vi "Whirlybird FPGA Main.vi"() -> (3 "Roll":i16)   [LabVIEW 2012]
uses:
  FPGA Samples/spi_single port_example/FPGA/Controls/FPGA SPI_Cmd.ctl
  <vilib>/Platform/TimedLoop/XDataNode/timing_clust.ctl
  <vilib>/Platform/TimedLoop/XDataNode/nitl_modes.ctl
  <vilib>/Platform/TimedLoop/XDataNode/wakeup.ctl
  FPGA Samples/spi_single port_example/FPGA/Controls/FPGA SPI_Arb Loop State.ctl
  <vilib>/rvi/eio/common/nirviEmuTemplateMethod_errors.vi
  <vilib>/rvi/Emulation/niFpgaSctlEmulationGetInTimedLoop.vi
  <vilib>/rvi/Emulation/niFpgaSctlEmulationGlobalWrite.vi
  FPGA Samples/spi_single port_example/FPGA/Code/FPGA SPI_Globals.vi
  <vilib>/rvi/DataTransferAndStorage/Container/Common/niFpgaContainerGetUniqueNameForEmu.vi
  <vilib>/rvi/FIFO/Fifo_Resource/nirvififoEmulationSetSize.vi
  <vilib>/rvi/errors/niFpgaSetErrorForExecOnDevCompSimple.vi
  <vilib>/rvi/eio/common/nirviEmuReportErrorAndStop.vi
  <vilib>/rvi/Emulation/niFpgaSctlEmulationFifoFullMgr.vi
  <vilib>/rvi/Emulation/niFpgaSctlEmulationResourceMgr.vi
  <vilib>/rvi/Emulation/niFpgaSctlEmulationRegisterWithScheduler.vi
  <vilib>/rvi/Emulation/niFpgaSctlEmulationScheduler.vi
  <vilib>/Platform/TimedLoop/XDataNode/XDataNode.xnode
  <vilib>/eio/EIONode/EIONode.xnode
  <vilib>/eio/EIOMethodNode/EIOMethodNode.xnode
  <vilib>/rvi/DataTransferAndStorage/Container/XNode/niFpgaContainer.xnode
  <vilib>/rvi/FIFO/Fifo_Resource/nirvififoEmulationWrite.vi
  <vilib>/rvi/FIFO/Fifo_Resource/nirvififoEmulationRead.vi
  <vilib>/Platform/TimedLoop/XDataNode/XDNodeRunTimeDep.lvlib
panel:
  in  "Auto Zero?":bool
  in  "IMU Reset":bool=TRUE
  in  "SPI_Ack Read":bool
  out "SPI_Read Flag":bool
  out "SPI_Read Data":u8
  in  "SPI_Write Data":u8
  in  "SPI_Write Flag":bool
  in  "SPI_Total Bytes":u16=1
  in  "SPI_Total Bits":u16=8
  in  "SPI_CS":u8=1 format="%08b"
  in  "SPI_CS Active State":bool caption="SPI_CS\nActive State"
  in  "SPI_Clock Divider":u32=20
  in  "SPI_CPHA":bool
  in  "SPI_CPOL":bool
  in  "SPI_Cmd":T1=enum."Configure"
  in  "SPI_Port":u8
  in  "SPI_Start":bool
  out "Ready":bool
  in  "MC2":u32(slide)=20 step=546002432 scale=0.0..600.0
  in  "MC1":u32(slide)=20 scale=0.0..600.0
  out "Pitch":i16
  out "Yaw":i16
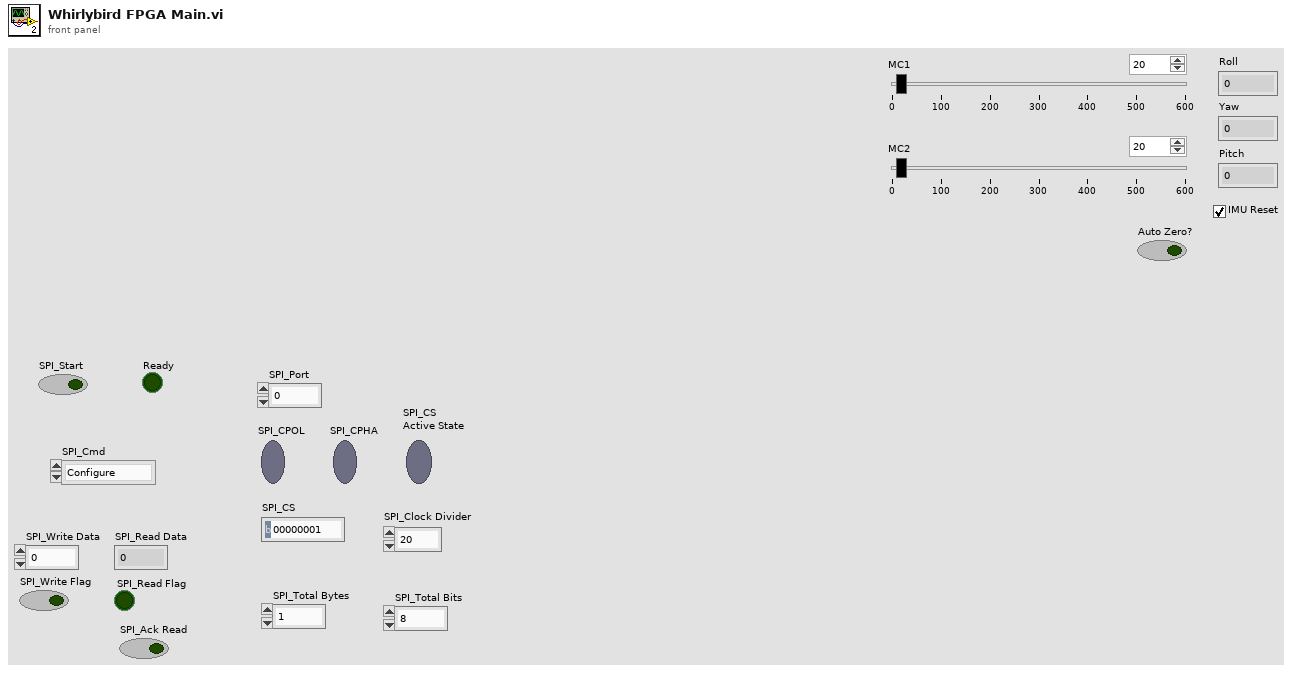
[diagram p1: front panel]
types:
  T1 = typedef "FPGA SPI_Cmd.ctl" = enum8{"Idle", "Write/Read SPI", "Configure"}
  T2 = cluster{"SCLK":refnum<k21>, "CS_1":refnum<k21>, "MOSI":refnum<k21>, "MISO":refnum<k21>, "CS_2":refnum<k21>}
  T3 = typedef "FPGA SPI_Arb Loop State.ctl" = enum8{"Idle", "Init", "Write", "Start", "Read", "Wait Until Done"}
  T4 = typedef "XDNodeRunTimeDep.lvlib/timing_clust.ctl" = cluster{"Expected End [f-1]":u64, "Actual End [f-1]":u64, "Finished Late? [f-1]":bool, "Expected End [i-1]":u64, "Actual End [i-1]":u64, "Finished Late? [i-1]":bool, "Expected Start [i]":u64, "Actual Start [i]":u64, "Expected Start [f]":u64, "Actual Start [f]":u64, "Source Name":string, "Structure Name":string, "Period":i64, "Deadline":i64, "Offset":i64, "Start":i64, "Priority":i32, "Timeout":i32, "Mode":T5, "Wakeup Reason":T6, "Error":errorcluster, "Source Type":string, "Secondary Source Type":string, "Global End Time":u64, "Global Start Time":u64, "Frame Duration":u64, "Iteration Duration":u64, "Assigned CPU":i32, "I/O Scan Engine Mode":u32}
  T5 = typedef "XDNodeRunTimeDep.lvlib/nitl_modes.ctl" = enum32{"No Change", "Process missed periods, maintain original phase", "Discard missed periods, maintain original phase", "Process missed periods, ignore original phase", "Discard missed periods, ignore original phase"}
  T6 = typedef "XDNodeRunTimeDep.lvlib/wakeup.ctl" = enum32{"Normal", "Aborted", "Asynchronous wakeup", "Timing source error", "Timed loop error", "Timeout"}
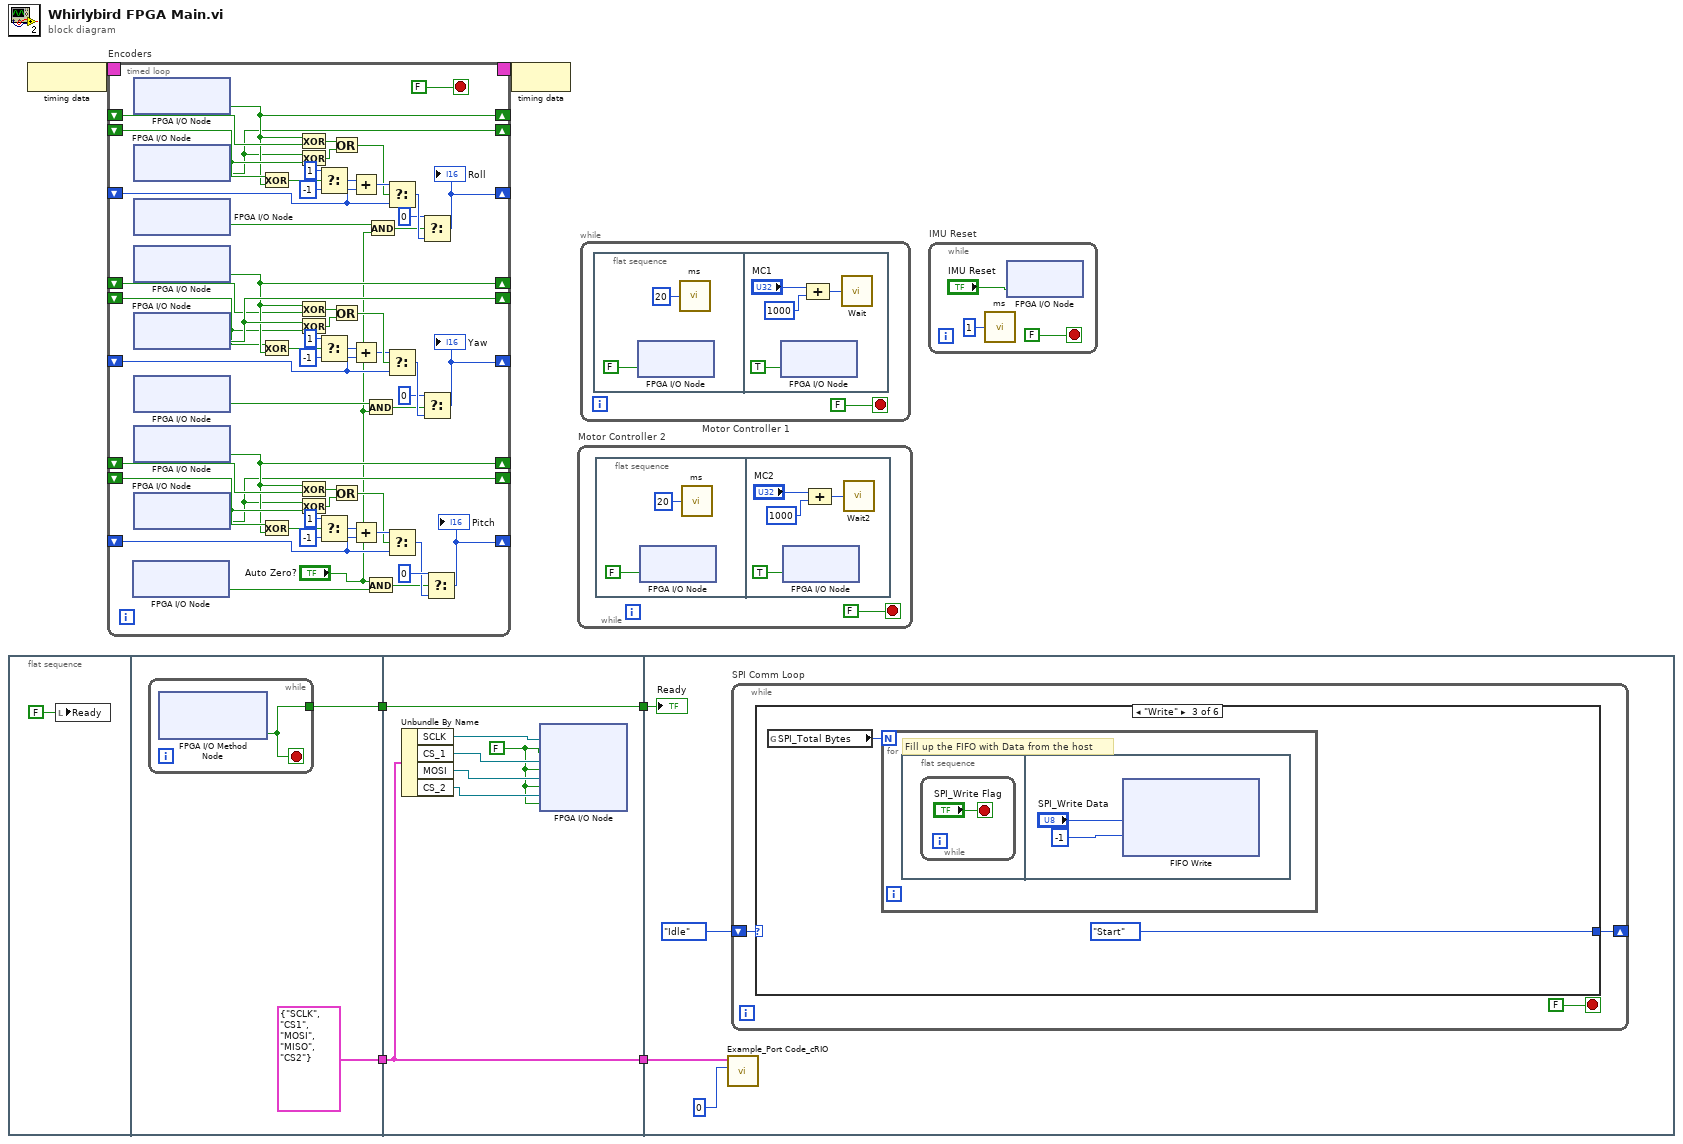
[diagram p0: block diagram]
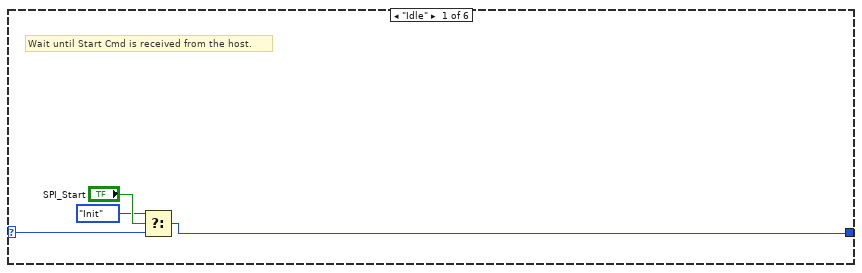
[diagram p2: hidden frame]
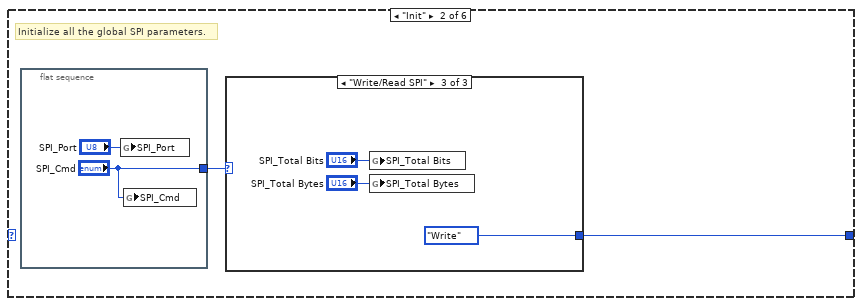
[diagram p3: hidden frame]
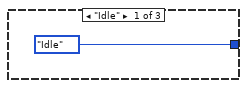
[diagram p4: hidden frame]
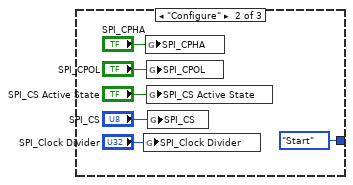
[diagram p5: hidden frame]
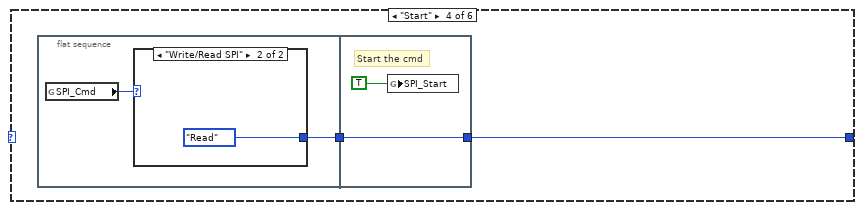
[diagram p6: hidden frame]
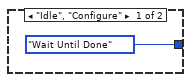
[diagram p7: hidden frame]
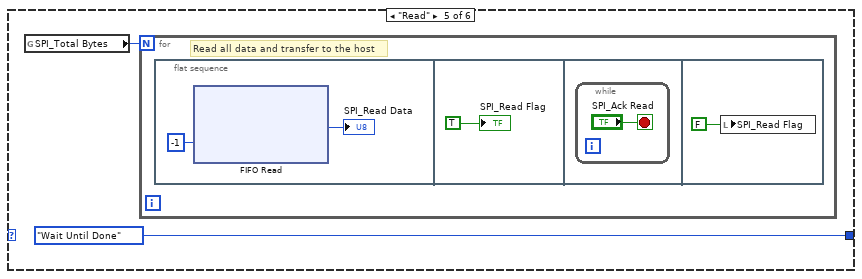
[diagram p8: hidden frame]
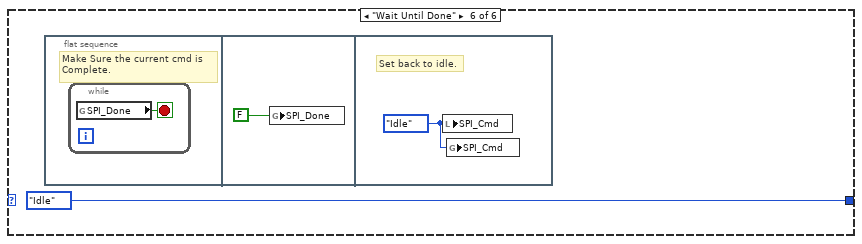
[diagram p9: hidden frame]
diagram:
  n1 = flat-sequence {
    tunnel: [T2 {"SCLK"="SCLK", "CS_1"="CS1", "MOSI"="MOSI", "MISO"="MISO", "CS_2"="CS2"} ("FPGA IO")] -> w4
    tunnel: [w8] -> w3
    tunnel: [w17] -> w2
    tunnel: w4 -> [w17]
    tunnel: [w13] -> w1
    tunnel: w3 -> [w13]
    tunnel: w2 -> [w19]
    tunnel: w1 -> [w18]
    frame #0 {
      n2 = local write "Ready"(FALSE ("Ready")) -> ()
    }
    frame #1 {
      n3 = while {
        tunnel: [w10] -> w8
        stop <- w10 stop-if-true
        n4 = xnode "FPGA I/O Method Node"() -> ("Ready"=w10:bool)  [unwired: 1 in, 1 out]
      }
    }
    frame #2 {
      w11 = FALSE ("I/O Item")
      n5 = Unbundle By Name(w17) -> ("SCLK"=w12:refnum<k21>, "CS_1"=w16:refnum<k21>, "MOSI"=w15:refnum<k21>, "CS_2"=w14:refnum<k21>)
      n6 = xnode "FPGA I/O Node"("I/O Item"=w11, "FPGA I/O In"=w12, "I/O Item"=w11, "FPGA I/O In"=w16, "I/O Item"=w11, "FPGA I/O In"=w15, "I/O Item"=w11, "FPGA I/O In"=w14) -> ()  [unwired: 4 out]
    }
    frame #3 {
      n7 = call "Example_Port Code_cRIO.vi"("Port"=i8 0, "FPGA IO"=w19) -> ()  [unwired: 10 out]
      n8 = while "SPI Comm Loop" {
        shift-right: [w23] -> _
        shift-left: FPGA_SPI_Arb_Loop_State."Idle" ("Action") -> [w22]
        stop <- FALSE stop-if-true
        n9 = case shown="\"Write\"" w22 {
          selector: w22 -> [w27 _ _ _ _ _]
          tunnel: [w25 w29 FPGA_SPI_Arb_Loop_State."Start" ("Action") w49 FPGA_SPI_Arb_Loop_State."Wait Until Done" ("Action") FPGA_SPI_Arb_Loop_State."Idle" ("Action")] -> w23
          frame "Idle" {
            # "Wait until Start Cmd is received from the host."
            n10 = Select(t=FPGA_SPI_Arb_Loop_State."Init" ("Action"), s="SPI_Start", f=w27) -> (s? t:f=w25:T3)
          }
          frame "Init" {
            # "Initialize all the global SPI parameters."
            n11 = flat-sequence {
              tunnel: ["SPI_Cmd"] -> w30
              frame #0 {
                n12 = global write "FPGA SPI_Globals.vi" "SPI_Port"("SPI_Port") -> ()
                n13 = global write "FPGA SPI_Globals.vi" "SPI_Cmd"("SPI_Cmd") -> ()
              }
            }
            n14 = case shown="\"Write/Read SPI\"" w30 {
              tunnel: [FPGA_SPI_Arb_Loop_State."Idle" ("Action") FPGA_SPI_Arb_Loop_State."Start" ("Action") FPGA_SPI_Arb_Loop_State."Write" ("Action")] -> w29
              frame "Idle" {
              }
              frame "Configure" {
                n15 = global write "FPGA SPI_Globals.vi" "SPI_Clock Divider"("SPI_Clock Divider") -> ()
                n16 = global write "FPGA SPI_Globals.vi" "SPI_CPHA"("SPI_CPHA") -> ()
                n17 = global write "FPGA SPI_Globals.vi" "SPI_CPOL"("SPI_CPOL") -> ()
                n18 = global write "FPGA SPI_Globals.vi" "SPI_CS Active State"("SPI_CS Active State") -> ()
                n19 = global write "FPGA SPI_Globals.vi" "SPI_CS"("SPI_CS") -> ()
              }
              frame "Write/Read SPI" {
                n20 = global write "FPGA SPI_Globals.vi" "SPI_Total Bits"("SPI_Total Bits") -> ()
                n21 = global write "FPGA SPI_Globals.vi" "SPI_Total Bytes"("SPI_Total Bytes") -> ()
              }
            }
          }
          frame "Write" {
            n22 = global read "FPGA SPI_Globals.vi" "SPI_Total Bytes"() -> (w44:u16)
            n23 = for {
              N: w44 -> [_]
              # "Fill up the FIFO with Data from the host"
              n24 = flat-sequence {
                frame #0 {
                  n25 = while {
                    stop <- "SPI_Write Flag" stop-if-true
                  }
                }
                frame #1 {
                  n26 = xnode ("FIFO Write")("Element"="SPI_Write Data", "Timeout"=-1) -> ()  [unwired: 1 in, 2 out]
                }
              }
            }
          }
          frame "Start" {
            n27 = flat-sequence {
              tunnel: [w50] -> w48
              tunnel: [w55] -> w49
              tunnel: w48 -> [w55]
              frame #0 {
                n28 = global read "FPGA SPI_Globals.vi" "SPI_Cmd"() -> (w51:T1)
                n29 = case shown="\"Write/Read SPI\"" w51 {
                  tunnel: [FPGA_SPI_Arb_Loop_State."Wait Until Done" ("Action") FPGA_SPI_Arb_Loop_State."Read" ("Action")] -> w50
                  frame "Idle", "Configure" {
                  }
                  frame "Write/Read SPI" {
                  }
                }
              }
              frame #1 {
                # "Start the cmd"
                n30 = global write "FPGA SPI_Globals.vi" "SPI_Start"(TRUE ("Write Flag")) -> ()
              }
            }
          }
          frame "Read" {
            n31 = global read "FPGA SPI_Globals.vi" "SPI_Total Bytes"() -> (w57:u16)
            n32 = for {
              N: w57 -> [_]
              # "Read all data and transfer to the host"
              n33 = flat-sequence {
                frame #0 {
                  n34 = xnode ("FIFO Read")("Timeout"=-1) -> ("Element"=→"SPI_Read Data":u8)  [unwired: 1 in, 2 out]
                }
                frame #1 {
                  "SPI_Read Flag" <- TRUE ("Read Flag")
                }
                frame #2 {
                  n35 = while {
                    stop <- "SPI_Ack Read" stop-if-true
                  }
                }
                frame #3 {
                  n36 = local write "SPI_Read Flag"(FALSE ("Read Flag")) -> ()
                }
              }
            }
          }
          frame "Wait Until Done" {
            n37 = flat-sequence {
              frame #0 {
                # "Make Sure the current cmd is\nComplete."
                n38 = while {
                  stop <- w64 stop-if-true
                  n39 = global read "FPGA SPI_Globals.vi" "SPI_Done"() -> (w64:bool)
                }
              }
              frame #1 {
                n40 = global write "FPGA SPI_Globals.vi" "SPI_Done"(FALSE ("Done")) -> ()
              }
              frame #2 {
                w66 = FPGA_SPI_Cmd."Idle" ("Type")
                # "Set back to idle."
                n41 = local write "SPI_Cmd"(w66) -> ()
                n42 = global write "FPGA SPI_Globals.vi" "SPI_Cmd"(w66) -> ()
              }
            }
          }
        }
      }
      "Ready" <- w18
    }
  }
  n43 = node-c288() -> (w6:T4)
  n44 = timed-loop "Encoders" {
    timing-out: [_] -> w5
    timing: w6 -> [_]
    shift-left: _ -> [w116]
    shift-right: [w110] -> _
    shift-left: _ -> [w112]
    shift-right: [w81] -> _
    shift-left: _ -> [w113]
    shift-right: [w111] -> _
    shift-right: [w108] -> _
    shift-left: _ -> [w102]
    shift-right: [w78] -> _
    shift-left: _ -> [w106]
    shift-right: [w107] -> _
    shift-left: _ -> [w105]
    shift-right: [w83] -> _
    shift-left: _ -> [w89]
    shift-right: [w74] -> _
    shift-left: _ -> [w85]
    shift-right: [w84] -> _
    shift-left: _ -> [w86]
    stop <- FALSE stop-if-true
    n45 = xnode "FPGA I/O Node"() -> ("Mod2/DI2"=w72:bool)  [unwired: 1 in, 1 out]
    n46 = xnode "FPGA I/O Node"() -> ("Mod1/DI0"=w111:bool)  [unwired: 1 in, 1 out]
    n47 = xnode "FPGA I/O Node"() -> ("Mod1/DI1"=w110:bool)  [unwired: 1 in, 1 out]
    n48 = xnode "FPGA I/O Node"() -> ("Mod1/DI2"=w69:bool)  [unwired: 1 in, 1 out]
    n49 = xnode "FPGA I/O Node"() -> ("Mod1/DI3"=w107:bool)  [unwired: 1 in, 1 out]
    n50 = xnode "FPGA I/O Node"() -> ("Mod1/DI4"=w108:bool)  [unwired: 1 in, 1 out]
    n51 = xnode "FPGA I/O Node"() -> ("Mod1/DI5"=w68:bool)  [unwired: 1 in, 1 out]
    n52 = xnode "FPGA I/O Node"() -> ("Mod2/DI0"=w84:bool)  [unwired: 1 in, 1 out]
    n53 = xnode "FPGA I/O Node"() -> ("Mod2/DI1"=w83:bool)  [unwired: 1 in, 1 out]
    n54 = Exclusive Or(1:w111, 2:w116) -> (0:w114:bool)
    n55 = Exclusive Or(1:w107, 2:w102) -> (0:w104:bool)
    n56 = Exclusive Or(1:w84, 2:w89) -> (0:w87:bool)
    n57 = Exclusive Or(1:w113, 2:w111) -> (0:w117:bool)
    n58 = Exclusive Or(1:w116, 2:w110) -> (0:w118:bool)
    n59 = Exclusive Or(1:w105, 2:w107) -> (0:w101:bool)
    n60 = Exclusive Or(1:w102, 2:w108) -> (0:w100:bool)
    n61 = Exclusive Or(1:w86, 2:w84) -> (0:w90:bool)
    n62 = Exclusive Or(1:w89, 2:w83) -> (0:w91:bool)
    n63 = Select(t=i16 1 ("16 bit"), s=w114, f=i16 -1 ("16 bit")) -> (s? t:f=w121:i16)
    n64 = Select(t=i16 1 ("16 bit"), s=w104, f=i16 -1 ("16 bit")) -> (s? t:f=w97:i16)
    n65 = Select(t=i16 1 ("16 bit"), s=w87, f=i16 -1 ("16 bit")) -> (s? t:f=w94:i16)
    n66 = Or(x=w117, y=w118) -> (x .or. y?=w115:bool)
    n67 = Or(x=w101, y=w100) -> (x .or. y?=w103:bool)
    n68 = Or(x=w90, y=w91) -> (x .or. y?=w88:bool)
    n69 = Add(x=w121, y=w112) -> (x+y=w122:i16)
    n70 = Add(x=w97, y=w106) -> (x+y=w96:i16)
    n71 = Add(x=w94, y=w85) -> (x+y=w95:i16)
    n72 = And(x=w68, y="Auto Zero?") -> (x .and. y?=w71:bool)
    n73 = And(x="Auto Zero?", y=w72) -> (x .and. y?=w73:bool)
    n74 = And(x=w69, y="Auto Zero?") -> (x .and. y?=w70:bool)
    n75 = Select(t=w122, s=w115, f=w112) -> (s? t:f=w82:i16)
    n76 = Select(t=w96, s=w103, f=w106) -> (s? t:f=w79:i16)
    n77 = Select(t=w95, s=w88, f=w85) -> (s? t:f=w75:i16)
    n78 = Select(t=i16 0, s=w70, f=w82) -> (s? t:f=w81:i16)
    "Roll" <- w81
    n79 = Select(t=i16 0, s=w71, f=w79) -> (s? t:f=w78:i16)
    "Yaw" <- w78
    n80 = Select(t=i16 0, s=w73, f=w75) -> (s? t:f=w74:i16)
    "Pitch" <- w74
  }
  n81 = node-c288(w5) -> ()
  n82 = while "Motor Controller 2" {
    stop <- FALSE stop-if-true
    n83 = flat-sequence {
      frame #0 {
        n84 = xnode "FPGA I/O Node"("MC2"=FALSE ("I2CSDA")) -> ()  [unwired: 1 in, 1 out]
        n85 = call "ms"("Count(mSec)"=u32 20 ("Count(uSec)")) -> ()  [unwired: 1 out]
      }
      frame #1 {
        n86 = xnode "FPGA I/O Node"("MC2"=TRUE ("I2CSDA")) -> ()  [unwired: 1 in, 1 out]
        n87 = Compound Arithmetic op=ADD("MC2", u32 1000 ("value")) -> (w129:u32)
        n88 = call "Wait2"("Count(uSec)"=w129) -> ()  [unwired: 1 out]
      }
    }
  }
  n89 = while "Motor Controller 1" {
    stop <- FALSE stop-if-true
    n90 = flat-sequence {
      frame #0 {
        n91 = xnode "FPGA I/O Node"("MC1"=FALSE ("I2CSDA")) -> ()  [unwired: 1 in, 1 out]
        n92 = call "ms"("Count(mSec)"=u32 20 ("Count(uSec)")) -> ()  [unwired: 1 out]
      }
      frame #1 {
        n93 = xnode "FPGA I/O Node"("MC1"=TRUE ("I2CSDA")) -> ()  [unwired: 1 in, 1 out]
        n94 = Compound Arithmetic op=ADD("MC1", u32 1000 ("value")) -> (w136:u32)
        n95 = call "Wait"("Count(uSec)"=w136) -> ()  [unwired: 1 out]
      }
    }
  }
  n96 = while "IMU Reset" {
    stop <- FALSE stop-if-true
    n97 = call "ms"("Count(mSec)"=u32 1 ("Count(uSec)")) -> ()  [unwired: 1 out]
    n98 = xnode "FPGA I/O Node"("Reset"="IMU Reset") -> ()  [unwired: 1 in, 1 out]
  }
